vi "LogBuffers.vi"(0 "Buffers in":T1={"Channels"=[], "PosttriggerBuffer"=refnum, "PretriggerBuffer"=refnum, "BlockSizePerChannel"=0, " logging semaphore"=refnum, "Log refnum"=refnum, "snapshotBuffer"=refnum, "logDirectory"=path "", "logPrefix"="", "decimation factor"=1, "max files"=0, "SampleRate"=0.0}, 7 "numOfChannels":i32, 11 "error in (no error)":errorcluster) -> (4 "Buffers out":T1={"Channels"=[], "PosttriggerBuffer"=refnum, "PretriggerBuffer"=refnum, "BlockSizePerChannel"=0, " logging semaphore"=refnum, "Log refnum"=refnum, "snapshotBuffer"=refnum, "logDirectory"=path "", "logPrefix"="", "decimation factor"=1, "max files"=0, "SampleRate"=0.0}, 15 "error out":errorcluster)   [LabVIEW 2017, in "BufferLogging.lvlib"]
uses:
  BufferLogging.lvlib
  Buffers.ctl
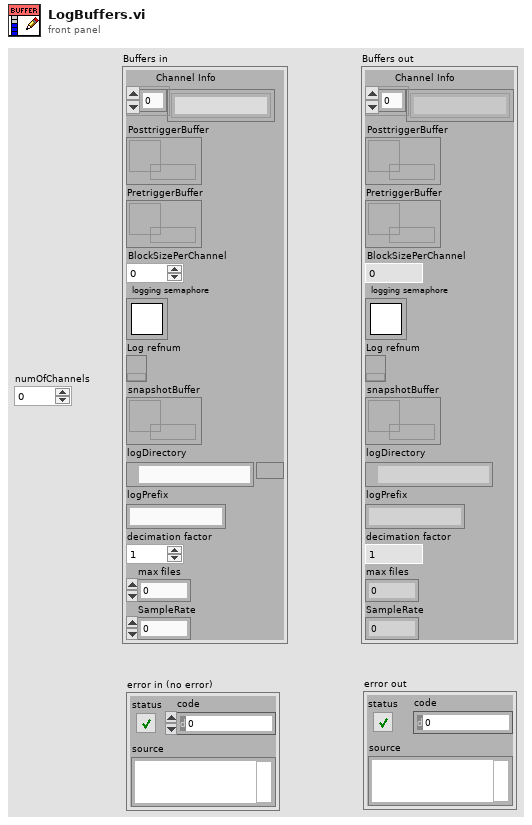
[diagram p1: front panel]
types:
  T1 = typedef "BufferLogging.lvlib/Buffers.ctl" = cluster{"Channels":string[], "PosttriggerBuffer":refnum<queue>, "PretriggerBuffer":refnum<queue>, "BlockSizePerChannel":i32, " logging semaphore":T2, "Log refnum":refnum<k34>, "snapshotBuffer":refnum<data-value>, "logDirectory":path, "logPrefix":string, "decimation factor":i32, "max files":i32, "SampleRate":dbl}
  T2 = typedef "Semaphore RefNum" = refnum<k1>
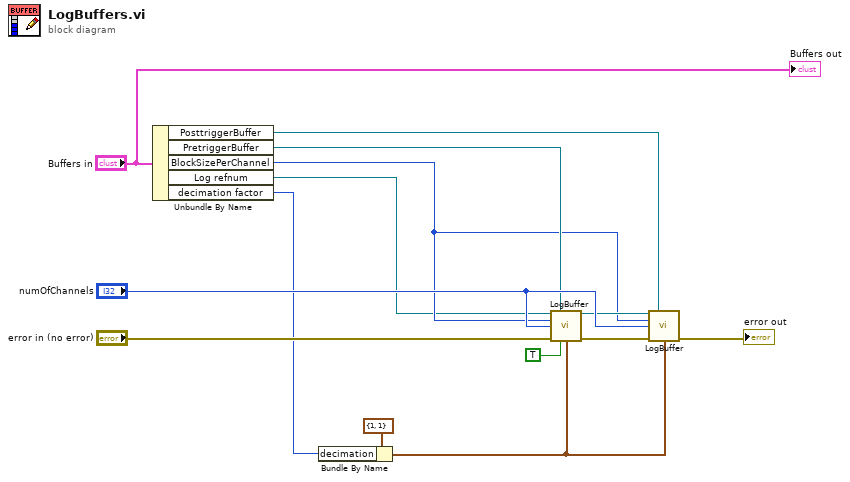
[diagram p0: block diagram]
diagram:
  n1 = Unbundle By Name("Buffers in") -> ("PosttriggerBuffer"=w7:refnum<queue>, "PretriggerBuffer"=w8:refnum<queue>, "BlockSizePerChannel"=w6:i32, "Log refnum"=w5:refnum<k34>, "decimation factor"=w1:i32)
  n2 = Bundle By Name(cluster=cluster{"interpolation":i32, "decimation":i32} {"interpolation"=1, "decimation"=1} ("resample factor"), "decimation"=w1) -> (w3:cluster{"interpolation":i32, "decimation":i32})
  n3 = call "LogBuffer.vi"("tdms file in"=w5, "Buffer in"=w8, "sizeOfBlock"=w6, "NumOfChannels"="numOfChannels", "error in (no error)"="error in (no error)", "resetResample"=TRUE ("resetOnFirstCall"), "resample factor"=w3) -> ("tdms file out"=w11:refnum<k34>, "error out"=w10:errorcluster)  [unwired: 7 in]
  n4 = call "LogBuffer.vi"("tdms file in"=w11, "Buffer in"=w7, "sizeOfBlock"=w6, "NumOfChannels"="numOfChannels", "error in (no error)"=w10, "resample factor"=w3) -> ("error out"=→"error out":errorcluster)  [unwired: 8 in, 1 out]
  "Buffers out" <- "Buffers in"
